vi "SetOutput.vi"(8 "error in (no error)":errorcluster, 11 "Laser Diode Controller in":refnum<class "KLD101.lvclass">) -> (0 "error out":errorcluster, 3 "Laser Diode Controller out":refnum<class "KLD101.lvclass">)   [LabVIEW 2016, in "Laser Diode Controller.lvlib" / "KLD101.lvclass"]
uses:
  KLD101.lvclass
  KLD101.lvclass/KLD101.ctl
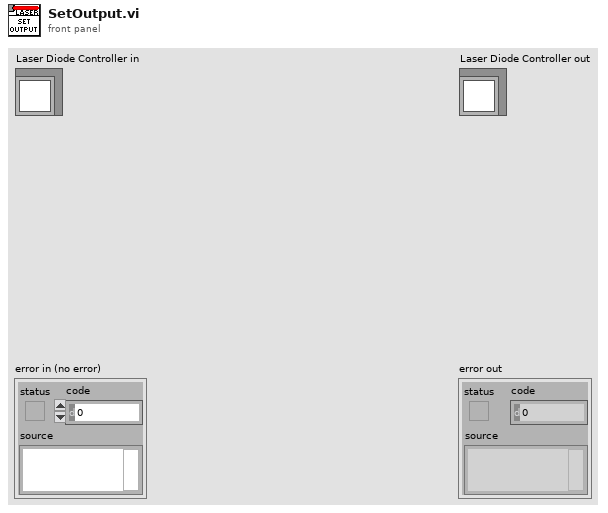
[diagram p1: front panel]
types:
  T1 = typedef "Laser Diode Controller.lvlib/KLD101.lvclass/KLD-LaserMode.ctl" = enum16{"Constant Power", "Constant Current"}
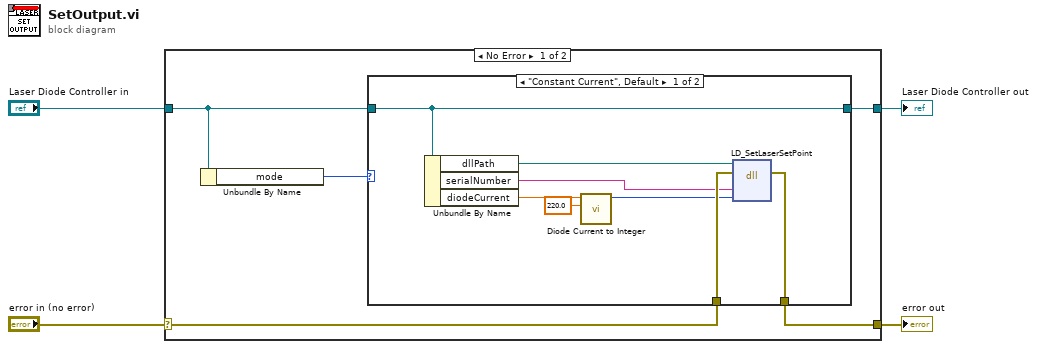
[diagram p0: block diagram]
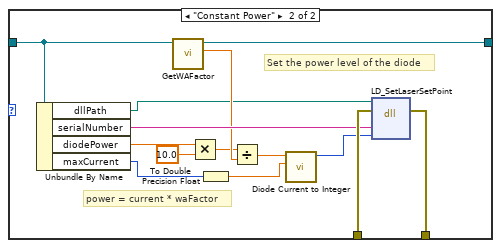
[diagram p2: hidden frame]
diagram:
  n1 = case shown="No Error" "error in (no error)" {
    selector: "error in (no error)" -> [w9 w33]
    tunnel: [w8 w33] -> w3
    tunnel: [w7 w32] -> w1
    tunnel: "Laser Diode Controller in" -> [w6 w32]
    frame No Error {
      n2 = Unbundle By Name(w6) -> ("mode"=w5:T1)
      n3 = case shown="\"Constant Current\", Default" w5 {
        tunnel: w9 -> [w17 w30]
        tunnel: [w16 w29] -> w8
        tunnel: w6 -> [w15 w27]
        tunnel: [w15 w26] -> w7
        frame "Constant Current", Default {
          n4 = Unbundle By Name(w15) -> ("dllPath"=w14:path, "serialNumber"=w13:string, "diodeCurrent"=w12:dbl)
          n5 = call "Diode Current to Integer.vi"("Max Current (mA)"=220.0, "Current (mA)"=w12) -> ("Current Int"=w10:i16)  [unwired: 9 in]
          n6 = dll-call lib="C:/IDEXX Software/Collimation/data/Thorlabs.MotionControl.KCube.LaserDiode.dll" fn="LD_SetLaserSetPoint"(path in=w14, error in=w17, "serialNumber"=w13, "laserDiodeCurrent"=w10) -> (error out=w16:errorcluster)  [unwired: 4 in, 1 out]
        }
        frame "Constant Power" {
          # "power = current * waFactor"
          # "Set the power level of the diode"
          n7 = Unbundle By Name(w27) -> ("dllPath"=w18:path, "serialNumber"=w28:string, "diodePower"=w31:dbl, "maxCurrent"=w20:i16)
          n8 = call-dynamic "GetWAFactor.vi"("Laser Diode Controller in"=w27) -> ("waFactor"=w25:dbl, "Laser Diode Controller out"=w26:refnum<class "KLD101.lvclass">)  [unwired: 8 in, 1 out]
          n9 = Multiply(x=w31, y=10.0) -> (x*y=w22:dbl)
          n10 = To Double Precision Float(number=w20) -> (double precision float=w19:dbl)
          n11 = Divide(x=w22, y=w25) -> (x/y=w24:dbl)
          n12 = call "Diode Current to Integer.vi"("Max Current (mA)"=w19, "Current (mA)"=w24) -> ("Current Int"=w23:i16)  [unwired: 9 in]
          n13 = dll-call lib="C:/IDEXX Software/Collimation/data/Thorlabs.MotionControl.KCube.LaserDiode.dll" fn="LD_SetLaserSetPoint"(path in=w18, error in=w30, "serialNumber"=w28, "laserDiodeCurrent"=w23) -> (error out=w29:errorcluster)  [unwired: 4 in, 1 out]
        }
      }
    }
    frame Error {
    }
  }
  "error out" <- w3
  "Laser Diode Controller out" <- w1
